vi "calculatePhase.vi"(1 "input":csg) -> (0 "output":dbl)   [LabVIEW 2023]
doc: "Purpose:\nThis VI calculates the phase (argument) of a given complex number in radians.\n\nInputs:\nComplex Number (complex): A complex number for which the phase is to be computed.\nOutputs:\nPhase (double): The phase of the complex number, calculated as theta = atan(Im/Re) where:\nRe is the real part\nIm is the imaginary part of the complex number.\n\nExecution Notes:\nThe output phase is in grad and lies in the range from -180 till 180\nMake sure the complex number is not purely real or imaginary for meaningful phase results."
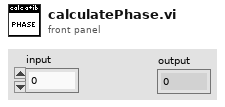
[diagram p1: front panel]
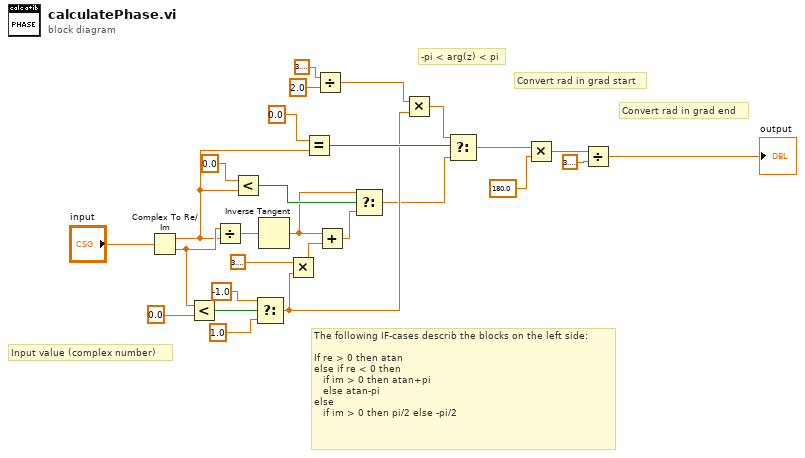
[diagram p0: block diagram]
diagram:
  # "Input value (complex number)"
  # "-pi < arg(z) < pi"
  # "The following IF-cases describ the blocks on the left side:\n\nIf re > 0 then atan \nelse if re < 0 then\n   if im > 0 then atan+pi\n   else atan-pi\nelse \n   if im > 0 then pi/2 else -pi/2"
  # "Convert rad in grad end"
  # "Convert rad in grad start"
  n1 = Complex To Re/Im(x + iy="input") -> (x=w11:sgl, y=w17:sgl)
  n2 = Less?(x=w17, y=0.0) -> (x < y?=w15:bool)
  n3 = Divide(x=w17, y=w11) -> (x/y=w18:sgl)
  n4 = Less?(x=0.0, y=w11) -> (x < y?=w10:bool)
  n5 = Select(t=-1.0, s=w15, f=1.0) -> (s? t:f=w7:dbl)
  n6 = Inverse Tangent(1:w18) -> (0:w9:sgl)
  n7 = Multiply(x=3.141592653589793, y=w7) -> (x*y=w6:dbl)
  n8 = Equal?(x=0.0, y=w11) -> (x = y?=w21:bool)
  n9 = Divide(x=3.141592653589793, y=2.0) -> (x/y=w4:dbl)
  n10 = Add(x=w9, y=w6) -> (x+y=w5:dbl)
  n11 = Select(t=w9, s=w10, f=w5) -> (s? t:f=w2:dbl)
  n12 = Multiply(x=w4, y=w7) -> (x*y=w3:dbl)
  n13 = Select(t=w3, s=w21, f=w2) -> (s? t:f=w1:dbl)
  n14 = Multiply(x=w1, y=180.0) -> (x*y=w26:dbl)
  n15 = Divide(x=w26, y=3.141592653589793) -> (x/y=→"output":dbl)
